vi "SaveDataVicon.vi"(7 "Array":dbl[][](array[numeric]), 9 "# of Expermintens":string, 10 "# of Version":string, 11 "Test Theme":string) -> (3 "File Name":string)   [LabVIEW 2017]
uses:
  <vilib>/Utility/file.llb/Write Delimited Spreadsheet (DBL).vi
  <vilib>/Utility/file.llb/Write Delimited Spreadsheet (string).vi
panel:
  in  "Array 2":string[](array[string])=["FF control", "Measured", "R1", "Deisred"]
  out "appended path":path
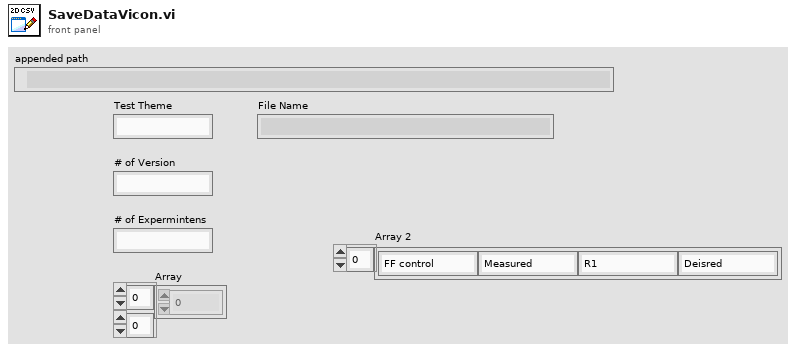
[diagram p1: front panel]
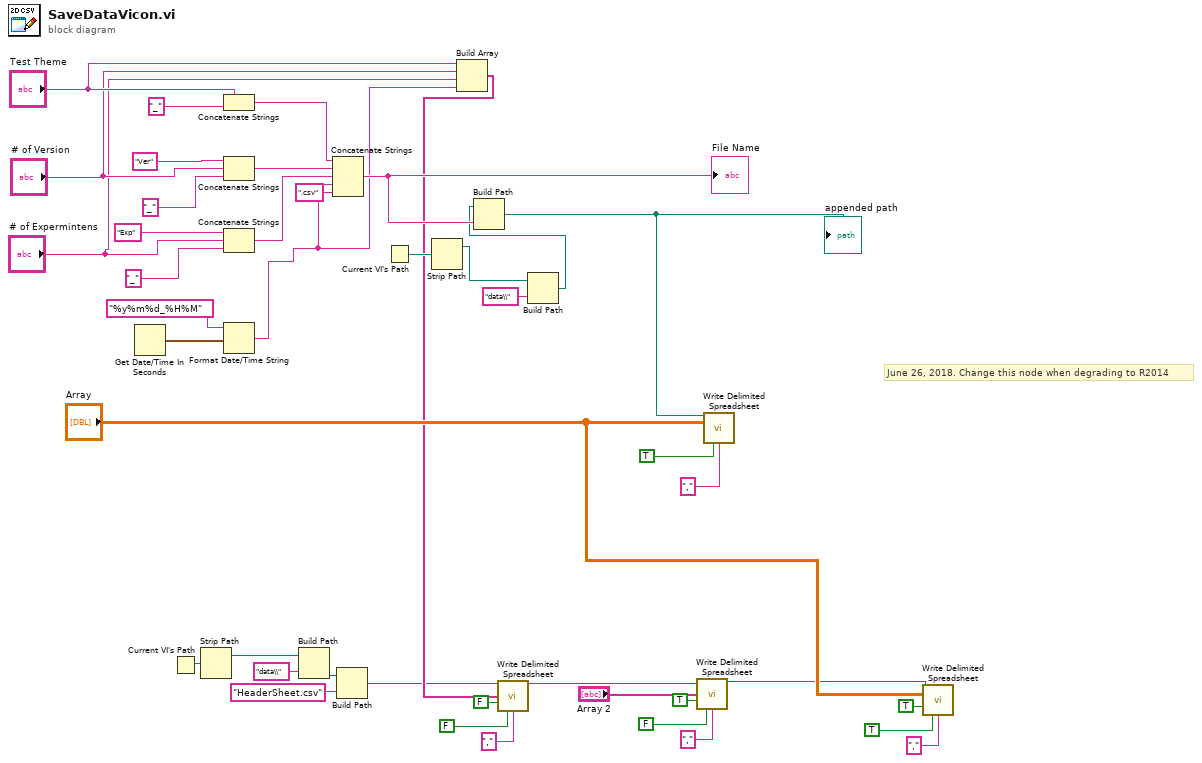
[diagram p0: block diagram]
diagram:
  # "June 26, 2018. Change this node when degrading to R2014"
  n1 = Get Date/Time In Seconds() -> (seconds since 1Jan1904=w29:timestamp)
  n2 = Current VI's Path() -> (path=w18:path)
  n3 = Strip Path(path=w18) -> (stripped path=w21:path)  [unwired: 1 out]
  n4 = Concatenate Strings("Test Theme", "_" ("string")) -> (w36:string)
  n5 = Concatenate Strings("Ver", "# of Version", "_" ("string")) -> (w39:string)
  n6 = Concatenate Strings("Exp", "# of Expermintens", "_" ("string")) -> (w38:string)
  n7 = Format Date/Time String(time format string (%c)="%y%m%d_%H%M", seconds (now)=w29) -> (date/time string=w4:string)  [unwired: 1 in]
  n8 = Build Path(base path=w21, name or relative path="data\\") -> (appended path=w20:path)
  n9 = Concatenate Strings(w36, w39, w38, w4, ".csv" ("string")) -> (w42:string)
  "File Name" <- w42
  n10 = Build Path(base path=w20, name or relative path="HeaderSheet.csv") -> (appended path=w2:path)
  n11 = Current VI's Path() -> (path=w28:path)
  n12 = Strip Path(path=w28) -> (stripped path=w22:path)  [unwired: 1 out]
  n13 = Build Array("Test Theme", "# of Version", "# of Expermintens", w4) -> (w3:string[])
  n14 = call-poly <vilib>:"Write Delimited Spreadsheet.vi"("file path (dialog if empty)"=w2, "1D data"=w3, "append to file? (new file:F)"=FALSE, "transpose? (no:F)"=FALSE, "delimiter (\\t)"="," ("delimiter (\\t)")) -> ("new file path (Not A Path if cancelled)"=w1:path)  [unwired: 9 in, 1 out]
  n15 = Build Path(base path=w22, name or relative path="data\\") -> (appended path=w26:path)
  n16 = Build Path(base path=w26, name or relative path=w42) -> (appended path=w43:path)
  "appended path" <- w43
  n17 = call-poly <vilib>:"Write Delimited Spreadsheet.vi"("file path (dialog if empty)"=w1, "1D data"="Array 2", "append to file? (new file:F)"=TRUE, "transpose? (no:F)"=FALSE, "delimiter (\\t)"="," ("delimiter (\\t)")) -> ("new file path (Not A Path if cancelled)"=w11:path)  [unwired: 9 in, 1 out]
  n18 = call-poly <vilib>:"Write Delimited Spreadsheet.vi"("file path (dialog if empty)"=w43, "2D data"="Array", "transpose? (no:F)"=TRUE, "delimiter (\\t)"="," ("delimiter (\\t)")) -> ()  [unwired: 10 in, 2 out]
  n19 = call-poly <vilib>:"Write Delimited Spreadsheet.vi"("file path (dialog if empty)"=w11, "2D data"="Array", "append to file? (new file:F)"=TRUE, "transpose? (no:F)"=TRUE, "delimiter (\\t)"="," ("delimiter (\\t)")) -> ()  [unwired: 9 in, 2 out]
